vi "RootFinder.vi"() -> ()   [LabVIEW 2024]
panel:
  out "x2":dbl
  out "x1":dbl
  in  "c":dbl
  in  "b":dbl
  in  "a":dbl
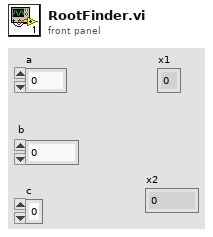
[diagram p1: front panel]
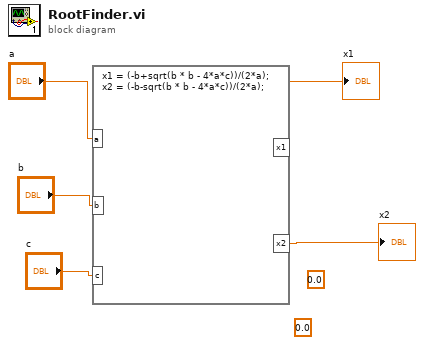
[diagram p0: block diagram]
diagram:
  (unwired) 0.0 ("Numeric")
  (unwired) 0.0 ("Numeric")
  n1 = formula code="x1 = (-b+sqrt(b * b - 4*a*c))/(2*a);\nx2 = (-b-sqrt(b * b - 4*a*c))/(2*a);"("a"="a", "b"="b", "c"="c") -> ("x2"=→"x2":dbl, "x1"=→"x1":dbl)
